vi "Waveform.vi"() -> ()   [LabVIEW 2018]
uses:
  Global.vi
panel:
  in  "Slide":dbl(slide) scale=0.0..10.0
  out "Waveform Chart":cluster{"Slider":dbl, "Knob":dbl}(graph)
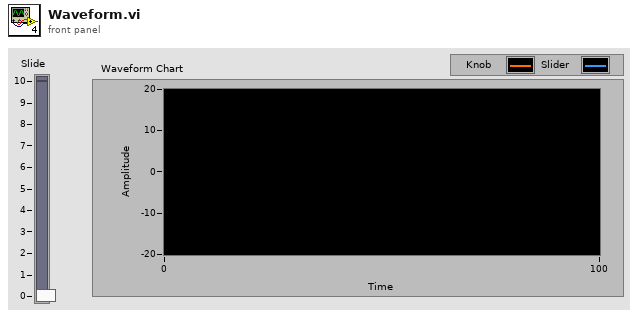
[diagram p1: front panel]
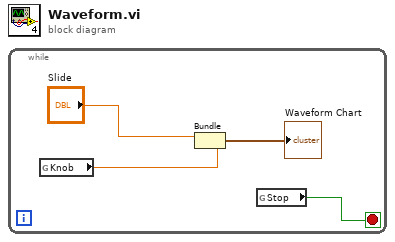
[diagram p0: block diagram]
diagram:
  n1 = while {
    stop <- w3 stop-if-true
    n2 = global read "Global.vi" "Knob"() -> (w2:dbl)
    n3 = Bundle("Slide"="Slide", "Knob"=w2) -> (→"Waveform Chart":cluster{"Slide":dbl, "Knob":dbl})  [unwired: 1 in]
    n4 = global read "Global.vi" "Stop"() -> (w3:bool)
  }
